vi "lvstyx_read_dir.vi"(2 "error in (no error)":errorcluster, 4 "path":string, 5 "client ptr":u32) -> (0 "error out":errorcluster, 1 "dir ptr":u32)   [LabVIEW 2010, in "lib1299.lvlib"]
uses:
  lib1299.lvlib
  cstyx/win32/cstyx.dll
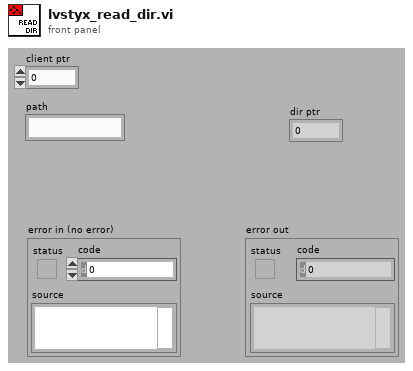
[diagram p1: front panel]
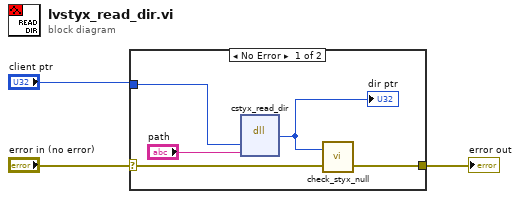
[diagram p0: block diagram]
diagram:
  n1 = case shown="No Error" "error in (no error)" {
    selector: "error in (no error)" -> [w6 w9]
    tunnel: "client ptr" -> [w7 _]
    tunnel: [w5 w9] -> w2
    frame No Error {
      n2 = dll-call lib="C:/work/ads1299evm/lib_1299/Styx/cstyx/win32/cstyx.dll" fn="cstyx_read_dir"("client"=w7, "path"="path") -> ("dir ptr"=w4:u32)  [unwired: 5 in, 2 out]
      "dir ptr" <- w4
      n3 = call "check_styx_null.vi"("error in (no error)"=w6, "ptr"=w4) -> ("error out"=w5:errorcluster)  [unwired: 3 in]
    }
    frame Error {
    }
  }
  "error out" <- w2
